vi "Approx Equal.vi"(2 "Tolerance":dbl, 3 "b":dbl, 4 "a":dbl) -> (0 "a-b":dbl, 1 "a == b?":bool)   [LabVIEW 2016]
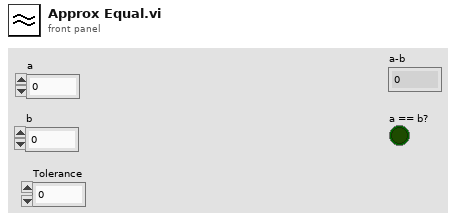
[diagram p1: front panel]
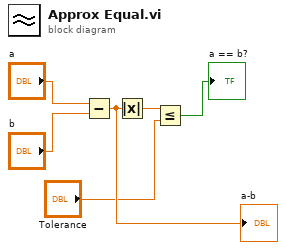
[diagram p0: block diagram]
diagram:
  n1 = Subtract(x="a", y="b") -> (x-y=w4:dbl)
  "a-b" <- w4
  n2 = Absolute Value(x=w4) -> (abs(x)=w3:dbl)
  n3 = Less Or Equal?(x=w3, y="Tolerance") -> (x <= y?=→"a == b?":bool)
